vi "FTW-Request-Receive.vi"(5 "Message":refnum<class "FTW-Message.lvclass">, 11 "error in":errorcluster) -> (4 "Initialized Request":refnum<class "FTW-Request.lvclass">, 6 "Request Header":string, 15 "error out":errorcluster)   [LabVIEW 2014, in "FTW-Request.lvclass"]
uses:
  FTW-Request.lvclass
  message/FTW-Message.lvclass
  FTW-Request.lvclass/FTW-Request.ctl
  error/FTW-ERR-ThrowError.vi
  error/FTW-ERR-CallChain.vi
  string/FTW-STR-ReplaceWhitespace.vi
  json/FTW-JSON.lvclass
panel:
  # "Inputs"
  # "Outputs"
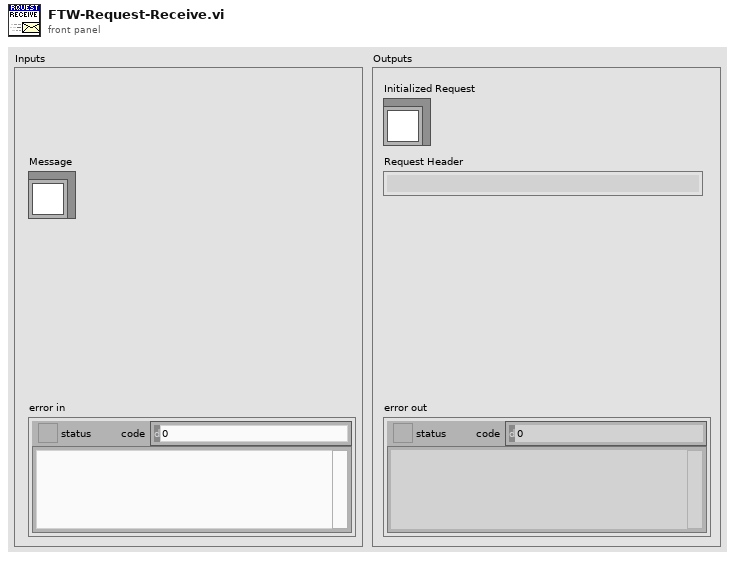
[diagram p1: front panel]
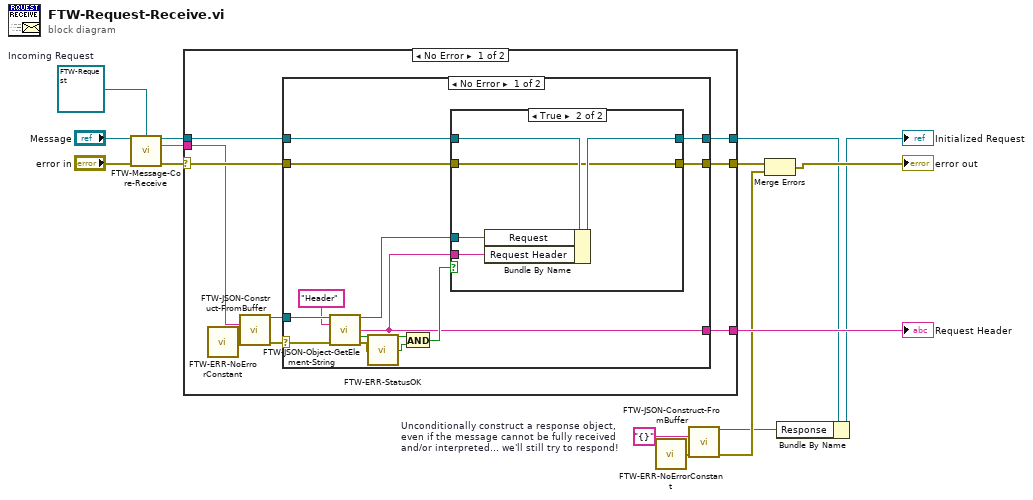
[diagram p0: block diagram]
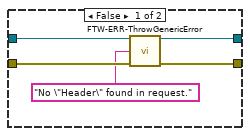
[diagram p2: hidden frame]
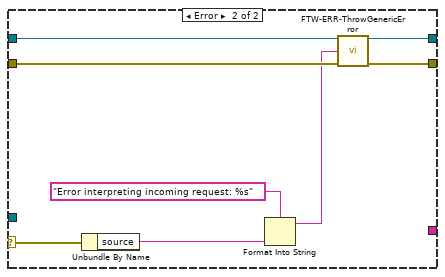
[diagram p3: hidden frame]
diagram:
  w8 = "{}"  # Unconditionally construct a response object, even if the message cannot be fully received and/or interpreted... we'll still try to respond!
  w12 = refnum<class "FTW-Request.lvclass"> refnum  # Incoming Request
  n1 = call "FTW-Message-Core-Receive.vi"("Incoming Message"="Message", "Expected Message Type"=w12, "error in"="error in") -> ("Constructed Message Type"=w11:refnum<class "FTW-Request.lvclass">, "Message"=w10:string, "error out"=w9:errorcluster)  [unwired: 10 in]
  n2 = case shown="No Error" w9 {
    selector: w9 -> [w18 w54]
    tunnel: [w22 w54] -> w6
    tunnel: [w21 _] -> w15
    tunnel: [w20 w55] -> w4
    tunnel: w11 -> [w19 w55]
    tunnel: w10 -> [w16 _]
    frame No Error {
      n3 = call "FTW-ERR-NoErrorConstant.vi"() -> ("no error"=w24:errorcluster)
      n4 = call "FTW-JSON-Construct-FromBuffer.vi"("JSON String (UTF-8)"=w16, "error in"=w24) -> ("JSON Object"=w23:refnum<class "FTW-JSON.lvclass">, "error out"=w17:errorcluster)  [unwired: 12 in]
      n5 = case shown="No Error" w17 {
        selector: w17 -> [w32 w48]
        tunnel: w23 -> [w37 _]
        tunnel: [w28 w51] -> w22
        tunnel: [w26 _] -> w21
        tunnel: [w34 w53] -> w20
        tunnel: w19 -> [w33 w53]
        tunnel: w18 -> [w27 w52]
        frame No Error {
          n6 = call "FTW-JSON-Object-GetElement-String.vi"("JSON Object"=w37, "Key"="Header", "error in"=w32) -> ("JSON Object out"=w36:refnum<class "FTW-JSON.lvclass">, "Value"=w26:string, "Found?"=w25:bool, "error out"=w31:errorcluster)  [unwired: 9 in]
          n7 = call "FTW-ERR-StatusOK.vi"("error to check"=w31) -> ("Status OK?"=w30:bool)
          n8 = And(x=w25, y=w30) -> (x .and. y?=w29:bool)
          n9 = case shown="True" w29 {
            tunnel: w36 -> [_ w46]
            tunnel: w26 -> [_ w45]
            tunnel: [w41 w44] -> w34
            tunnel: w33 -> [w41 w43]
            tunnel: [w39 w42] -> w28
            tunnel: w27 -> [w40 w42]
            frame False {
              n10 = call "FTW-ERR-ThrowGenericError.vi"("Error Message"="No \"Header\" found in request.", "error in"=w40) -> ("error out"=w39:errorcluster)  [unwired: 13 in]
            }
            frame True {
              n11 = Bundle By Name(cluster=w43, "Request"=w46, "Request Header"=w45) -> (w44:refnum<class "FTW-Request.lvclass">)
            }
          }
        }
        frame Error {
          n12 = Unbundle By Name(w48) -> ("source"=w47:string)
          n13 = Format Into String(format string="Error interpreting incoming request: %s", w47) -> (resulting string=w49:string)  [unwired: 2 in, 1 out]
          n14 = call "FTW-ERR-ThrowGenericError.vi"("Error Message"=w49, "error in"=w52) -> ("error out"=w51:errorcluster)  [unwired: 13 in]
        }
      }
    }
    frame Error {
    }
  }
  "Request Header" <- w15
  n15 = call "FTW-ERR-NoErrorConstant.vi"() -> ("no error"=w7:errorcluster)
  n16 = call "FTW-JSON-Construct-FromBuffer.vi"("JSON String (UTF-8)"=w8, "error in"=w7) -> ("JSON Object"=w3:refnum<class "FTW-JSON.lvclass">, "error out"=w5:errorcluster)  [unwired: 12 in]
  n17 = Merge Errors(w6, w5) -> (→"error out":errorcluster)
  n18 = Bundle By Name(cluster=w4, "Response"=w3) -> (→"Initialized Request":refnum<class "FTW-Request.lvclass">)
